vi "Usage IR Sensor.vi"() -> ()   [LabVIEW 2011, in "Wiimote.lvlib"]
uses:
  Wiimote.lvlib
  Wiimote Buttons.ctl
  Wiimote Acceleration.ctl
panel:
  in  "index":i32
  out "IR Sensor":cluster{"X":u16, "Y":u16}[](graph)
  out "Wiimote Acceleration out":T1
  out "Wiimote Buttons out":T2
  in  "stop":bool
  out "error out":errorcluster
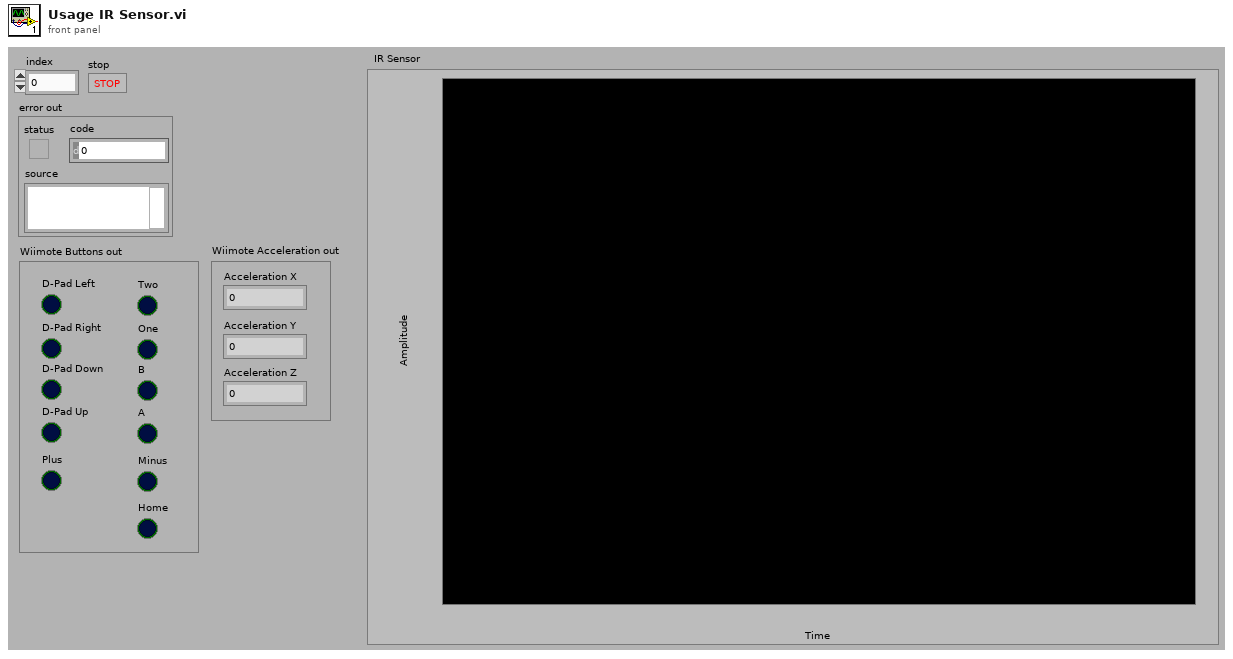
[diagram p1: front panel]
types:
  T1 = typedef "Wiimote.lvlib/Wiimote Acceleration.ctl" = cluster{"Acceleration X":dbl, "Acceleration Y":dbl, "Acceleration Z":dbl}
  T2 = typedef "Wiimote.lvlib/Wiimote Buttons.ctl" = cluster{"D-Pad Left":bool, "D-Pad Right":bool, "D-Pad Down":bool, "D-Pad Up":bool, "Plus":bool, "Two":bool, "One":bool, "B":bool, "A":bool, "Minus":bool, "Home":bool}
  T3 = typedef "Wiimote.lvlib/Wiimote IR Sensor.ctl" = cluster{"Point 1":T4, "Point 2":T4, "Point 3":T4, "Point 4":T4}
  T4 = typedef "Wiimote.lvlib/Wiimote Point.ctl" = cluster{"X":u16, "Y":u16}
  T5 = typedef "Wiimote.lvlib/Nunchuk Buttons.ctl" = cluster{"C":bool, "Z":bool}
  T6 = cluster{"Wiimote Buttons":T2, "Wiimote Acceleration Raw":T1, "Wiimote IR Sensor":T3, "Nunchuk Analog Stick":T4, "Nunchuk Acceleration Raw":T1, "Nunchuk Buttons":T5}
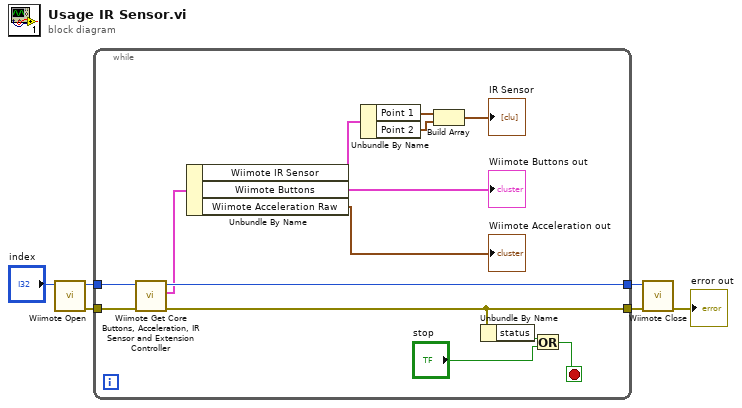
[diagram p0: block diagram]
diagram:
  n1 = call "Wiimote Open.vi"("index"="index") -> ("error out"=w2:errorcluster, "hWiimoteHandle"=w3:u32)  [unwired: 9 in]
  n2 = while {
    tunnel: w3 -> [w20]
    tunnel: w2 -> [w19]
    tunnel: [w18] -> w5
    tunnel: [w14] -> w4
    stop <- w11 stop-if-true
    n3 = call "Wiimote Get Core Buttons, Acceleration, IR Sensor and Extension Controller.vi"("error in"=w19, "hWiimoteHandle in"=w20) -> ("error out"=w14:errorcluster, "Data out"=w10:T6, "hWiimoteHandle out"=w18:u32)  [unwired: 7 in]
    n4 = Unbundle By Name(w10) -> ("Wiimote IR Sensor"=w9:T3, "Wiimote Buttons"=→"Wiimote Buttons out":T2, "Wiimote Acceleration Raw"=→"Wiimote Acceleration out":T1)
    n5 = Unbundle By Name(w9) -> ("Point 1"=w17:T4, "Point 2"=w16:T4)
    n6 = Build Array(w17, w16) -> (→"IR Sensor":T4[])
    n7 = Unbundle By Name(w14) -> ("status"=w13:bool)
    n8 = Or(x=w13, y="stop") -> (x .or. y?=w11:bool)
  }
  n9 = call "Wiimote Close.vi"("error in"=w4, "hWiimoteHandle in"=w5) -> ("error out"=→"error out":errorcluster)  [unwired: 9 in]
